vi "Get Destination Folder.vi"(8 "error in":errorcluster, 11 "User VI Ref":refnum<vi>) -> (0 "error out":errorcluster, 3 "Destination Folder":path)   [LabVIEW 2022 SP3]
doc: "Gets the Destination Folder location. This is the location where the new VI or CTL is going to be saved.\n\nNormally, the Destination Folder is the folder location that stores the User VI (the VI from which the user right-clicked to fire up the Shortcut Menu).\n\nOtherwise, the VI returns the User Desktop."
uses:
  <vilib>/Utility/sysdir.llb/System Directory Type.ctl
panel:
  out "User VI Path":path
  # "Development\ncontrols/indicators useful for development and testing, but which are not outputs of the VI"
  # "Input\nInputs to the VI"
  # "Output\nOutputs of the VI"
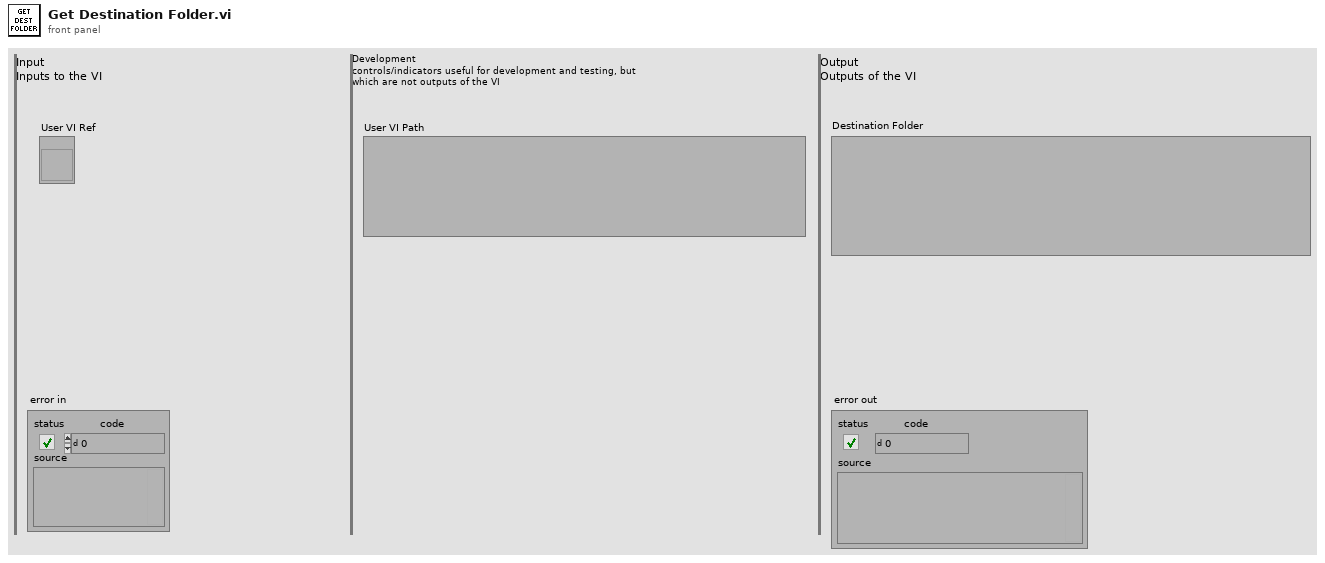
[diagram p1: front panel]
types:
  T1 = typedef "System Directory Type.ctl" = i32
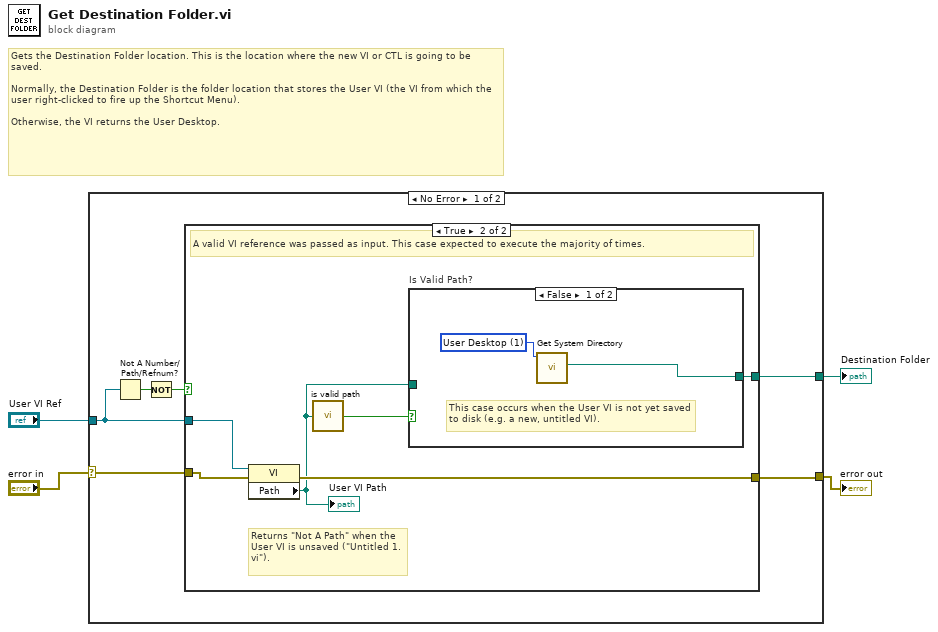
[diagram p0: block diagram]
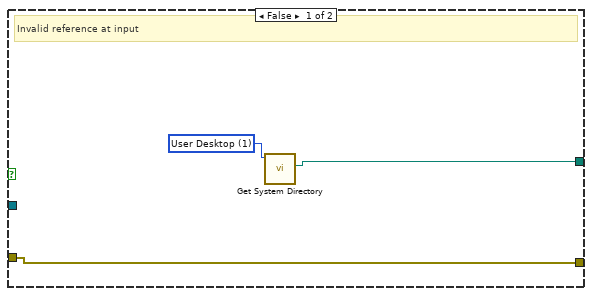
[diagram p2: hidden frame]
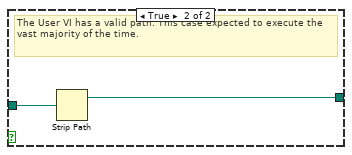
[diagram p3: hidden frame]
diagram:
  # "Gets the Destination Folder location. This is the location where the new VI or CTL is going to be saved.\n\nNormally, the Destination Folder is the folder location that stores the User VI (the VI from which the user right-clicked to fire up the Shortcut Menu).\n\nOtherwise, the VI returns the User Desktop."
  n1 = case shown="No Error" "error in" {
    selector: "error in" -> [w10 w24]
    tunnel: [w8 w24] -> w3
    tunnel: "User VI Ref" -> [w7 _]
    tunnel: [w9 _] -> w1
    frame No Error {
      n2 = Not A Number/Path/Refnum?(number/path/refnum=w7) -> (NaN/Path/Refnum?=w6:bool)
      n3 = Not(x=w6) -> (.not. x?=w5:bool)
      n4 = case shown="True" w5 {
        tunnel: w10 -> [w11 w19]
        tunnel: [w12 w18] -> w9
        tunnel: [w11 w17] -> w8
        tunnel: w7 -> [_ w16]
        frame False {
          w13 = T1 1 items=["User Home"=0, "User Desktop"=1, "User Documents"=2, "User Application Data"=3, "User Preferences"=4, "User Temporary"=5, "Public Documents"=6, "Public Application Data"=7, "Public Preferences"=8, "Public Cache"=13, "System Core Libraries"=9, "System Installed Libraries"=10, "Application Files"=11, "Boot Volume Root"=12] ("system directory type")
          # "Invalid reference at input"
          n5 = call <vilib>:"Get System Directory.vi"("system directory type"=w13) -> ("system directory"=w12:path)  [unwired: 10 in]
        }
        frame True {
          # "Returns \"Not A Path\" when the User VI is unsaved (\"Untitled 1.vi\")."
          # "A valid VI reference was passed as input. This case expected to execute the majority of times."
          n6 = property class="VI"(reference=w16, error in=w19) -> (error out=w17:errorcluster, "Path"=w15:path)  [unwired: 1 out]
          "User VI Path" <- w15
          n7 = call "is valid path.vi"("Path"=w15) -> ("Is valid path?"=w14:bool)
          n8 = case "Is Valid Path?" shown="False" w14 {
            tunnel: [w20 w22] -> w18
            tunnel: w15 -> [_ w23]
            frame False {
              w21 = T1 1 items=["User Home"=0, "User Desktop"=1, "User Documents"=2, "User Application Data"=3, "User Preferences"=4, "User Temporary"=5, "Public Documents"=6, "Public Application Data"=7, "Public Preferences"=8, "Public Cache"=13, "System Core Libraries"=9, "System Installed Libraries"=10, "Application Files"=11, "Boot Volume Root"=12] ("system directory type")
              # "This case occurs when the User VI is not yet saved to disk (e.g. a new, untitled VI)."
              n9 = call <vilib>:"Get System Directory.vi"("system directory type"=w21) -> ("system directory"=w20:path)  [unwired: 10 in]
            }
            frame True {
              # "The User VI has a valid path. This case expected to execute the vast majority of the time."
              n10 = Strip Path(path=w23) -> (stripped path=w22:path)  [unwired: 1 out]
            }
          }
        }
      }
    }
    frame Error {
    }
  }
  "error out" <- w3
  "Destination Folder" <- w1
